vi "Transit_Stdby_w_Lidlock.vi"(0 "GEA2 Reference In":refnum<k24>, 5 "Option Selection":T1, 7 "ECT Parameters":T2, 11 "Error In":errorcluster) -> (4 "GEA2 Reference Out":refnum<k24>, 6 "Machine State Pass/Fail":bool, 8 "Report text":string, 15 "Error Out":errorcluster)   [LabVIEW 2016, in "TL27.lvlib"]
doc: "This vi can be used to read ERD every 1 sec for user selected repeat counts."
uses:
  Projects/TL27.lvlib
  C:/Automation/DLLs/PC Dot Net/GeaCommunication.dll
  Controls/ECT Parameters.ctl
  Controls/Options.ctl
  Common/LabVIEW GEA2 Toolkit/LabVIEW_GEA2_Toolkit.lvlibp/type defs/Source_Destination.ctl
  Common/LabVIEW GEA2 Toolkit/LabVIEW_GEA2_Toolkit.lvlibp/type defs/ERD Read Data In.ctl
  Common/LabVIEW GEA2 Toolkit/LabVIEW_GEA2_Toolkit.lvlibp/type defs/Data Type.ctl
  Valew Common/type defs/Encoder Position.ctl
  Common/LabVIEW GEA2 Toolkit/LabVIEW_GEA2_Toolkit.lvlibp
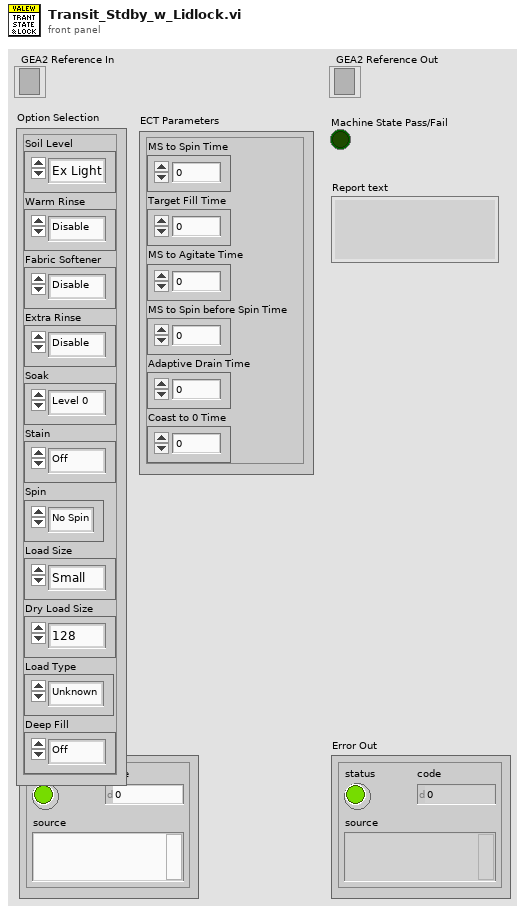
[diagram p1: front panel]
types:
  T1 = typedef "TL27.lvlib/Options.ctl" = cluster{"Soil Level":enum8{"Ex Light", "Light", "Normal", "Heavy", "Ex Heavy"}, "Warm Rinse":enum8{"Disable", "Enable"}, "Fabric Softener":enum16{"Disable", "Enable"}, "Extra Rinse":enum8{"Disable", "Enable"}, "Soak":enum8{"Level 0", "Level 1", "Level 2", "Level 3", "Level 4"}, "Stain":enum8{"Off", "Tomato", "Wine", "Blood", "Grass", "Dirt"}, "Spin":enum16{"No Spin", "Normal Spin", "More Spin", "Max Spin"}, "Load Size":enum8{"Small", "Medium", "Large", "Super", "Precise Fill", "Super Plus"}, "Dry Load Size":enum16{"128", "256", "384", "5AA", "6A4", "834", "65535"}, "Load Type":enum8{"Unknown", "Cotton", "Synthetic", "Mixed", "Wet", "Low Flow", "Small", "Medium", "Large", "Super", "Super Plus", "Max"}, "Deep Fill":enum8{"Off", "Incremental Fill", "Max Fill"}}
  T2 = typedef "TL27.lvlib/ECT Parameters.ctl" = cluster{"MS to Spin Time":u16, "Target Fill Time":u16, "MS to Agitate Time":u16, "MS to Spin before Spin Time ":u16, "Adaptive Drain Time":u16, "Coast to 0 Time":u16}
  T3 = typedef "LabVIEW_GEA2_Toolkit.lvlibp/Source_Destination.ctl" = cluster{"Source":u8, "Destination":u8}
  T4 = enum16{"EQ (==)", "NE (!=)", "GT (>)", "LT (<)", "GE (>=)", "LE (<=)", "GTLT(> <)", "GELE (>= <=)", "GELT (>= <)", "GTLE (> <=)", "LTGT (< >)", "LEGE (<= >=)", "LEGT (<= >)", "LTGE (< >=)", "No Comparison"}
  T5 = typedef "LabVIEW_GEA2_Toolkit.lvlibp/ERD Read Data In.ctl" = cluster{"ERD Number":u16, "Data Type":T6}
  T6 = typedef "LabVIEW_GEA2_Toolkit.lvlibp/Data Type.ctl" = enum16{"string", "boolean", "uint8_t", "uint16_t", "uint32_t", "uint64_t", "int8_t", "int16_t", "int32_t", "int64_t"}
  T7 = typedef "TL27.lvlib/Encoder Position.ctl" = enum16{"Position 0", "Position 1", "Position 2", "Position 3", "Position 4", "Position 5", "Position 6", "Position 7", "Position 8", "Position 9", "Position 10", "Position 11", "Position 12", "Position 13", "Clear / Reset"}
  T8 = typedef "TL27.lvlib/ECT.ctl" = cluster{"MS to Agitate Time":u16, "Adaptive Drain Time":u16, "Coast to 0 Time":u16, "Agitate Time":u16, "Warm Rinse Time":u16, "FS Time":u16, "Ex Rinse Time":u16, "Soak Time":u16, "Stain Time":u16, "Motor Profile ID":u16, "Calculated ECT":u16, "Spin Time":u16}
  T9 = typedef "LabVIEW_GEA2_Toolkit.lvlibp/ERD Read Data Out.ctl" = cluster{"ERD Number":u16, "Data":string}
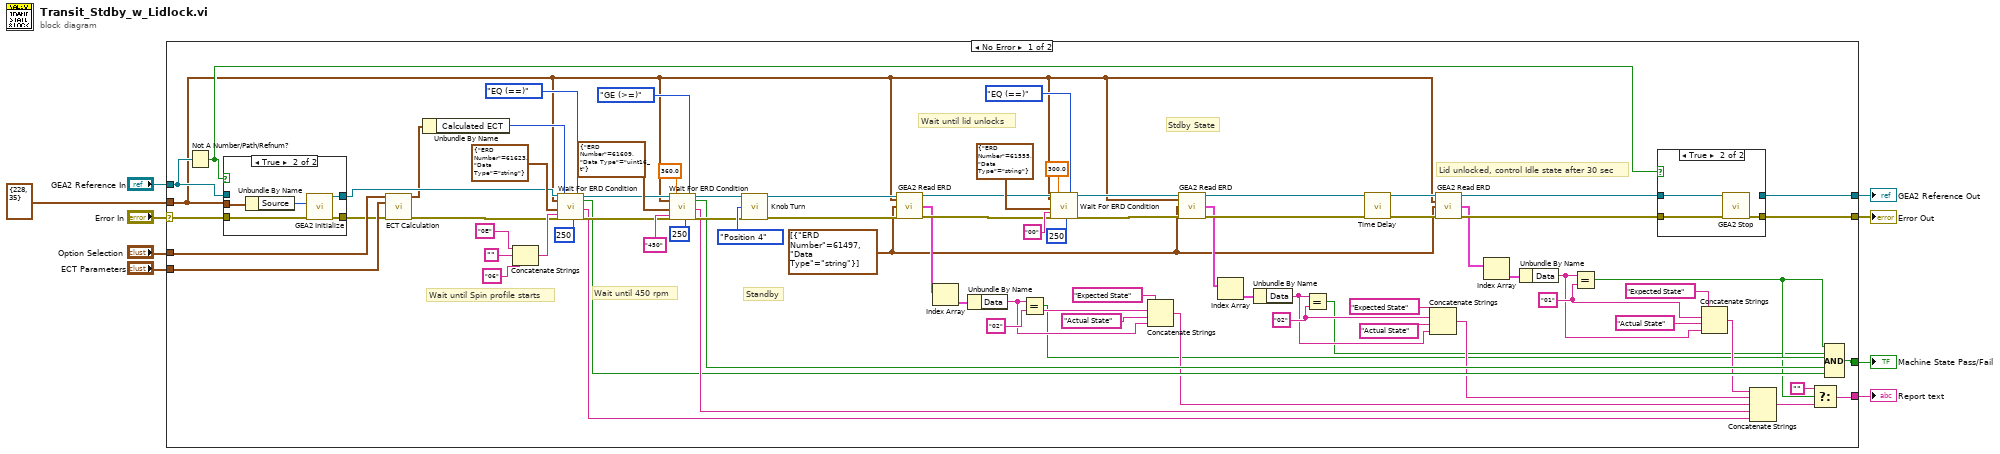
[diagram p0: block diagram]
diagram:
  n1 = case shown="No Error" "Error In" {
    selector: "Error In" -> [w87 w101]
    tunnel: T3 {"Source"=228, "Destination"=35} ("GEA Inputs") -> [w31 _]
    tunnel: "GEA2 Reference In" -> [w88 w102]
    tunnel: [w67 w102] -> w6
    tunnel: [w86 w101] -> w5
    tunnel: [w49 _] -> w4
    tunnel: [w59 _] -> w3
    tunnel: "Option Selection" -> [w14 _]
    tunnel: "ECT Parameters" -> [w13 _]
    frame No Error {
      w20 = "02" ("y")
      w26 = "02" ("y")
      w10 = T5[] [{"ERD Number"=61497, "Data Type"=enum."string"}] ("Read ERD List")
      w63 = "01" ("y")
      # "Stdby State"
      # "Wait until lid unlocks"
      # "Lid unlocked, control Idle state after 30 sec"
      # "Standby"
      # "Wait until 450 rpm"
      # "Wait until Spin profile starts"
      n2 = Not A Number/Path/Refnum?(number/path/refnum=w88) -> (NaN/Path/Refnum?=w85:bool)
      n3 = case shown="True" w85 {
        tunnel: w87 -> [w95 w100]
        tunnel: [w95 w99] -> w12
        tunnel: [w94 w98] -> w79
        tunnel: w31 -> [_ w96]
        tunnel: w88 -> [w94 _]
        frame False {
        }
        frame True {
          n4 = Unbundle By Name(w96) -> ("Source"=w97:u8)
          n5 = call "GEA2 Initialize.vi"("Source Address"=w97, "error in"=w100) -> ("GEA2 Reference Out"=w98:refnum<k24>, "error out"=w99:errorcluster)  [unwired: 11 in, 1 out]
        }
      }
      n6 = call "ECT Calculation.vi"("Option Selection"=w14, "ECT Parameters"=w13, "Error In"=w12) -> ("Expected ECT"=w55:T8, "Error Out"=w11:errorcluster)  [unwired: 11 in]
      n7 = Unbundle By Name(w55) -> ("Calculated ECT"=w66:u16)
      n8 = Concatenate Strings("0E" ("string"), "", "06" ("string")) -> (w82:string)
      n9 = call "Wait For ERD Condition.vi"("GEA2 Reference In"=w79, "GEA Inputs"=w31, "ERD Read Data"=T5 {"ERD Number"=61623, "Data Type"=enum."string"}, "Expected Low"=w82, "Error In"=w11, "Timeout (s)"=w66, "Loop Rate (ms)"=u32 250, "Comparison"=T4."EQ (==)") -> ("GEA2 Reference Out"=w73:refnum<k24>, "Pass/Fail?"=w52:bool, "Report Text"=w54:string, "Error Out"=w71:errorcluster)  [unwired: 7 in, 1 out]
      n10 = call "Wait For ERD Condition.vi"("GEA2 Reference In"=w73, "GEA Inputs"=w31, "ERD Read Data"=T5 {"ERD Number"=61609, "Data Type"=enum."uint16_t"}, "Expected Low"="450", "Error In"=w71, "Timeout (s)"=360.0, "Loop Rate (ms)"=u32 250, "Comparison"=T4."GE (>=)") -> ("GEA2 Reference Out"=w72:refnum<k24>, "Pass/Fail?"=w51:bool, "Report Text"=w53:string, "Error Out"=w70:errorcluster)  [unwired: 7 in, 1 out]
      n11 = call "Knob Turn.vi"("GEA2 Reference In"=w72, "Button"=Encoder_Position."Position 4", "Error In"=w70) -> ("GEA2 Reference Out"=w41:refnum<k24>, "Error Out"=w39:errorcluster)  [unwired: 11 in]
      n12 = call "GEA2 Read ERD.vi"("GEA2 Reference In"=w41, "GEA Inputs"=w31, "Read ERD List"=w10, "Error In"=w39) -> ("GEA2 Reference Out"=w40:refnum<k24>, "ERD Data Out"=w32:T9[], "Error Out"=w38:errorcluster)  [unwired: 8 in, 1 out]
      n13 = Index Array(array=w32) -> (element=w33:T9)  [unwired: 1 in]
      n14 = Unbundle By Name(w33) -> ("Data"=w25:string)
      n15 = Equal?(x=w25, y=w26) -> (x = y?=w17:bool)
      n16 = call "Wait For ERD Condition.vi"("GEA2 Reference In"=w40, "GEA Inputs"=w31, "ERD Read Data"=T5 {"ERD Number"=61555, "Data Type"=enum."string"}, "Expected Low"="00", "Error In"=w38, "Timeout (s)"=300.0, "Loop Rate (ms)"=u32 250, "Comparison"=T4."EQ (==)") -> ("GEA2 Reference Out"=w37:refnum<k24>, "Error Out"=w36:errorcluster)  [unwired: 7 in, 3 out]
      n17 = Concatenate Strings("Expected State" ("string"), w26, "Actual State" ("string"), w25) -> (w23:string)
      n18 = call "GEA2 Read ERD.vi"("GEA2 Reference In"=w37, "GEA Inputs"=w31, "Read ERD List"=w10, "Error In"=w36) -> ("GEA2 Reference Out"=w35:refnum<k24>, "ERD Data Out"=w29:T9[], "Error Out"=w34:errorcluster)  [unwired: 8 in, 1 out]
      n19 = Index Array(array=w29) -> (element=w30:T9)  [unwired: 1 in]
      n20 = Unbundle By Name(w30) -> ("Data"=w19:string)
      n21 = Equal?(x=w19, y=w20) -> (x = y?=w15:bool)
      n22 = call "Time Delay"("error in (no error)"=w34) -> ("error out"=w56:errorcluster)  [unwired: 10 in]
      n23 = Concatenate Strings("Expected State" ("string"), w20, "Actual State" ("string"), w19) -> (w18:string)
      n24 = call "GEA2 Read ERD.vi"("GEA2 Reference In"=w35, "GEA Inputs"=w31, "Read ERD List"=w10, "Error In"=w56) -> ("GEA2 Reference Out"=w69:refnum<k24>, "ERD Data Out"=w57:T9[], "Error Out"=w68:errorcluster)  [unwired: 8 in, 1 out]
      n25 = Index Array(array=w57) -> (element=w58:T9)  [unwired: 1 in]
      n26 = Unbundle By Name(w58) -> ("Data"=w61:string)
      n27 = Equal?(x=w61, y=w63) -> (x = y?=w16:bool)
      n28 = case shown="True" w85 {
        tunnel: [w89 w93] -> w86
        tunnel: w69 -> [w90 w92]
        tunnel: w68 -> [w89 w91]
        tunnel: [w90 _] -> w67
        frame False {
        }
        frame True {
          n29 = call "GEA2 Stop.vi"("GEA2 Reference In"=w92, "Error In"=w91) -> ("Error Out"=w93:errorcluster)  [unwired: 13 in]
        }
      }
      n30 = Concatenate Strings("Expected State" ("string"), w63, "Actual State" ("string"), w61) -> (w24:string)
      n31 = Concatenate Strings(w24, w18, w23, w53, w54) -> (w50:string)
      n32 = Select(t="", s=w16, f=w50) -> (s? t:f=w59:string)
      n33 = Compound Arithmetic op=AND(w16, w15, w17, w51, w52) -> (w49:bool)
    }
    frame Error {
    }
  }
  "GEA2 Reference Out" <- w6
  "Error Out" <- w5
  "Machine State Pass/Fail" <- w4
  "Report text" <- w3
